vi "rotate XY graf.vi"(10 "replased":cluster{timestamp[], dbl[]}[](array[cluster]), 11 "XY Graf in":cluster{timestamp[], dbl[]}[](array[cluster])) -> (3 "XY Graf out":cluster{timestamp[], dbl[]}[](array[cluster]))   [LabVIEW 2019]
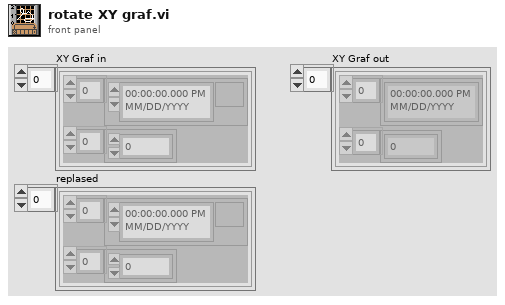
[diagram p1: front panel]
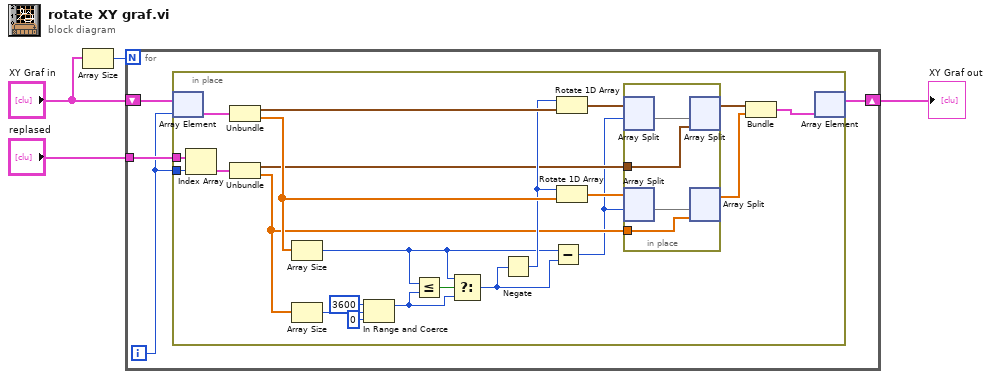
[diagram p0: block diagram]
diagram:
  n1 = Array Size(array="XY Graf in") -> (size(s)=w3:i32)
  n2 = for {
    N: w3 -> [_]
    tunnel: "replased" -> [w8]
    shift-right: [w5] -> w4
    shift-left: "XY Graf in" -> [w6]
    i -> [w7]
    n3 = in-place {
      in-place-border: w8 -> [w30]
      in-place-border: w7 -> [w29]
      n4 = in-place-array #1(w6, w7) -> (w20:cluster{timestamp[], dbl[]})
      n5 = Index Array(array=w30, index=w29) -> (element=w22:cluster{timestamp[], dbl[]})
      n6 = Unbundle(w20) -> (w28:timestamp[], w27:dbl[])
      n7 = Unbundle(w22) -> (w23:timestamp[], w17:dbl[])
      n8 = Array Size(array=w27) -> (size(s)=w13:i32)
      n9 = Array Size(array=w17) -> (size(s)=w10:i32)
      n10 = In Range and Coerce(upper limit=3600, x=w10, lower limit=0) -> (coerced(x)=w9:i32)  [unwired: 1 out]
      n11 = Less Or Equal?(x=w13, y=w9) -> (x <= y?=w26:bool)
      n12 = Select(t=w13, s=w26, f=w9) -> (s? t:f=w24:i32)
      n13 = Negate(x=w24) -> (-x=w25:i32)
      n14 = Subtract(x=w13, y=w24) -> (x-y=w14:i32)
      n15 = Rotate 1D Array(1:w28, 2:w25) -> (0:w19:timestamp[])
      n16 = Rotate 1D Array(1:w27, 2:w25) -> (0:w18:dbl[])
      n17 = in-place {
        in-place-border: w23 -> [w33]
        in-place-border: w17 -> [w32]
        n18 = in-place-split #2(w19, w14) -> (w34:timestamp[])  [unwired: 1 out]
        n19 = in-place-split #3(w18, w14) -> (w31:dbl[])  [unwired: 1 out]
        n20 = in-place-split #2(w34, w33) -> (w15:timestamp[])  [unwired: 1 out]
        n21 = in-place-split #3(w31, w32) -> (w16:dbl[])  [unwired: 1 out]
      }
      n22 = Bundle(w15, w16) -> (w21:cluster{timestamp[], dbl[]})  [unwired: 1 in]
      n23 = in-place-array #1(w21) -> (w5:cluster{timestamp[], dbl[]}[])  [unwired: 1 out]
    }
  }
  "XY Graf out" <- w4
